vi "Lookup Active Alarm By Code.vi"(10 "Code":i32, 11 "Active Alarms":T1[](array[typedef])) -> (2 "Index":i32, 3 "Found":bool)   [LabVIEW 2015, in "Alarm Handler Actor.lvclass"]
doc: "Searches through the Active Alarms for the alarm specified by <b>Code</b>."
uses:
  Alarm Handler Actor.lvclass
  Active Alarm.ctl
  Alarm Details.ctl
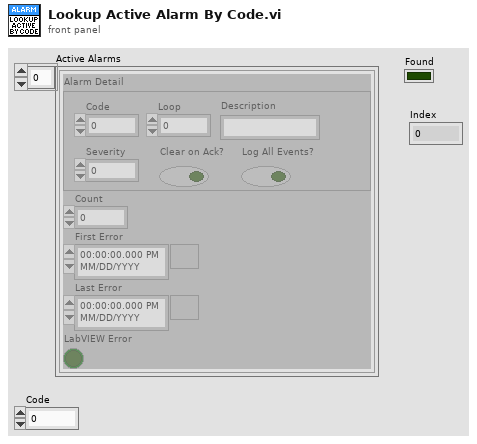
[diagram p1: front panel]
types:
  T1 = typedef "Alarm Handler Actor.lvclass/Active Alarm.ctl" = cluster{"Alarm Detail":T2, "Count":i32, "First Error":timestamp, "Last Error":timestamp, "LabVIEW Error":bool}
  T2 = typedef "Alarm Handler Actor.lvclass/Alarm Details.ctl" = cluster{"Code":i32, "Loop":i32, "Description":string, "Severity":i32, "Clear on Ack?":bool, "Log All Events?":bool}
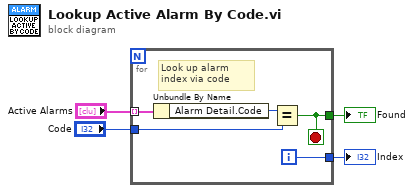
[diagram p0: block diagram]
diagram:
  n1 = for {
    tunnel: "Active Alarms" -> [w9] mode=indexing
    tunnel: "Code" -> [w7]
    tunnel: [w6] -> w2
    tunnel: [w5] -> w4
    i -> [w5]
    stop <- w6 stop-if-true
    # "Look up alarm index via code"
    n2 = Unbundle By Name(w9) -> ("Alarm Detail.Code"=w8:i32)
    n3 = Equal?(x=w8, y=w7) -> (x = y?=w6:bool)
  }
  "Index" <- w4
  "Found" <- w2
